vi "Write String.vi"(7 "Bus In":refnum<class "Bus.lvclass">, 8 "error in (no error)":errorcluster, 9 "Values":dbl[](array[numeric]), 10 "Data String":string, 11 "NI Digital in":refnum<class "NI Analog Out.lvclass">) -> (0 "error out":errorcluster, 2 "Bus Out":refnum<class "Bus.lvclass">, 3 "NI Digital out":refnum<class "NI Analog Out.lvclass">)   [LabVIEW 2018, in "NI Analog Out.lvclass"]
doc: "Bus.lvclass:Read String.vi\n\nThis is the template for the Read String VI forthe Bus class.\n\nInstrument Communication Module Version 1.0\nJuly, 2017 Original Code Consulting David Thomson\n www.originalcode.com"
uses:
  NI Analog Out.lvclass
  Bus/Bus.lvclass
  NI Analog Out.lvclass/NI Analog Out.ctl
  <vilib>/DAQmx/write.llb/DAQmx Write (Analog 1D DBL NChan 1Samp).vi
  <vilib>/DAQmx/miscellaneous.llb/DAQmx Fill In Error Info.vi
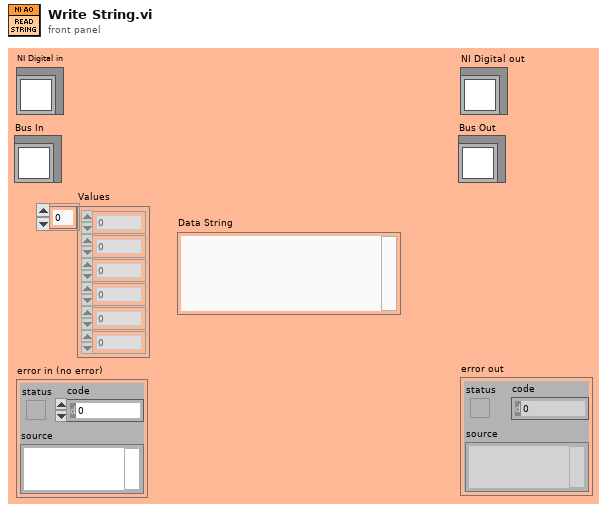
[diagram p1: front panel]
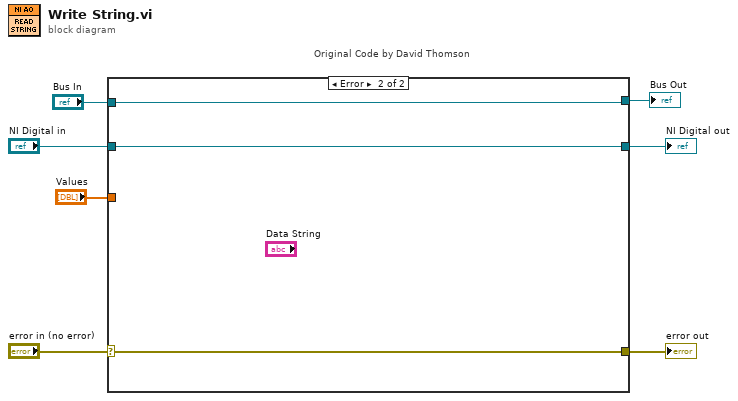
[diagram p0: block diagram]
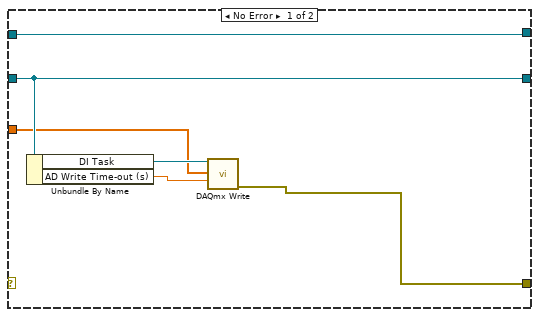
[diagram p2: hidden frame]
diagram:
  n1 = case "Original Code by David Thomson" shown="Error" "error in (no error)" {
    selector: "error in (no error)" -> [_ w16]
    tunnel: [w9 w16] -> w6
    tunnel: [w12 w15] -> w5
    tunnel: "NI Digital in" -> [w12 w15]
    tunnel: "Values" -> [w10 _]
    tunnel: "Bus In" -> [w8 w14]
    tunnel: [w8 w14] -> w1
    frame No Error {
      n2 = Unbundle By Name(w12) -> ("DI Task"=w13:refnum<k21>, "AD Write Time-out (s)"=w11:dbl)
      n3 = call-poly <vilib>:"DAQmx Write.vi"("task/channels in"=w13, "data"=w10, "timeout"=w11) -> ("error out"=w9:errorcluster)  [unwired: 10 in, 2 out]
    }
    frame Error {
    }
  }
  "error out" <- w6
  "NI Digital out" <- w5
  "Bus Out" <- w1
